vi "olcmeson.vi"() -> ()   [LabVIEW 2018]
panel:
  out "?":bool
  out "?":bool
  out "?":bool
  out "Aydınlık Seviyesi":bool
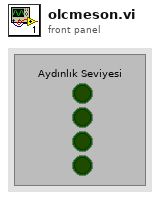
[diagram p1: front panel]
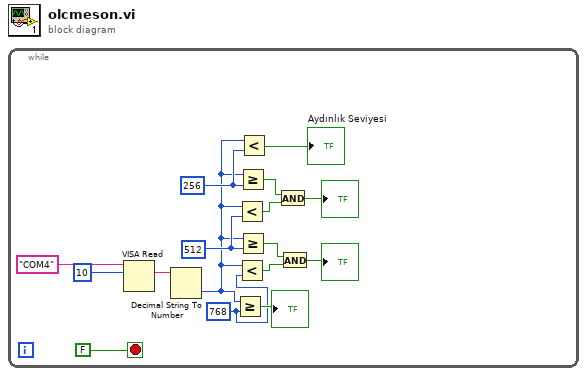
[diagram p0: block diagram]
diagram:
  n1 = while {
    stop <- FALSE stop-if-true
    w3 = 256
    w7 = 512
    w11 = 768
    n2 = VISA Read(VISA resource name="COM4", byte count=10) -> (read buffer=w13:string)  [unwired: 1 in, 3 out]
    n3 = Decimal String To Number(string=w13) -> (number=w2:i32)  [unwired: 2 in, 1 out]
    n4 = Greater Or Equal?(x=w2, y=w11) -> (x >= y?=→"?":bool)
    n5 = Less?(x=w2, y=w7) -> (x < y?=w5:bool)
    n6 = Less?(x=w2, y=w11) -> (x < y?=w10:bool)
    n7 = Greater Or Equal?(x=w2, y=w3) -> (x >= y?=w6:bool)
    n8 = Greater Or Equal?(x=w2, y=w7) -> (x >= y?=w9:bool)
    n9 = Less?(x=w2, y=w3) -> (x < y?=→"Aydınlık Seviyesi":bool)
    n10 = And(x=w6, y=w5) -> (x .and. y?=→"?":bool)
    n11 = And(x=w9, y=w10) -> (x .and. y?=→"?":bool)
  }
